vi "test open previous test.vi"() -> ()   [LabVIEW 2019]
panel:
  out "standard error":string
  out "standard output":string
  out "error out":errorcluster
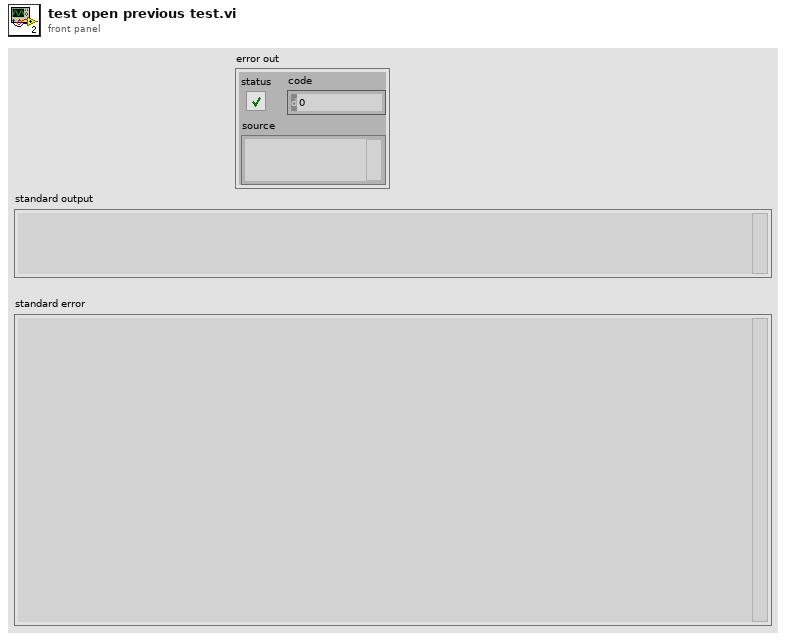
[diagram p1: front panel]
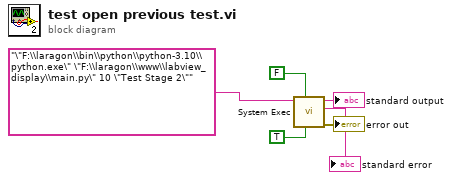
[diagram p0: block diagram]
diagram:
  n1 = call <vilib>:"System Exec.vi"("run minimized? (F)"=TRUE, "wait until completion? (T)"=FALSE, "command line"="\"F:\\laragon\\bin\\python\\python-3.10\\python.exe\" \"F:\\laragon\\www\\labview_display\\main.py\" 10 \"Test Stage 2\"") -> ("error out"=→"error out":errorcluster, "standard error"=→"standard error":string, "standard output"=→"standard output":string)  [unwired: 5 in, 1 out]
